vi "Init.vi"(7 "Round":u32, 8 "error in (no error)":errorcluster, 9 "Team In":refnum<class "Team.lvclass">, 10 "Board Size":i32, 11 "Square in":refnum<class "Square.lvclass">) -> (0 "error out":errorcluster, 1 "Team":refnum<class "Team.lvclass">, 3 "Square out":refnum<class "Square.lvclass">)   [LabVIEW 2020, in "SquareBattle.lvlib" / "Square.lvclass"]
uses:
  Square.lvclass
  Team/Team.lvclass
  Square.lvclass/Square.ctl
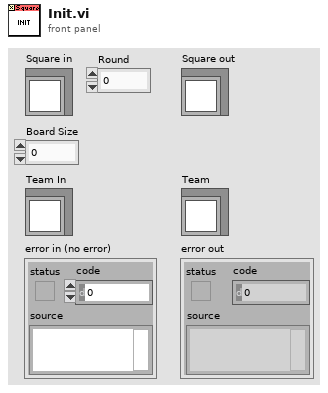
[diagram p1: front panel]
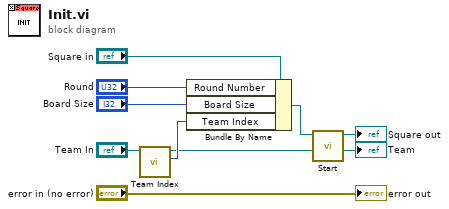
[diagram p0: block diagram]
diagram:
  n1 = call "Team Index.vi"("Team in"="Team In") -> ("Team Index"=w6:i32, "Team out"=w4:refnum<class "Team.lvclass">)  [unwired: 8 in, 1 out]
  n2 = Bundle By Name(cluster="Square in", "Round Number"="Round", "Board Size"="Board Size", "Team Index"=w6) -> (w5:refnum<class "Square.lvclass">)
  n3 = call-dynamic "Start.vi"("Team In"=w4, "Square in"=w5) -> ("Team"=→"Team":refnum<class "Team.lvclass">, "Square out"=→"Square out":refnum<class "Square.lvclass">)  [unwired: 8 in]
  "error out" <- "error in (no error)"
